vi "get filter mode.vi"(10 "filter rate":dbl, 11 "Numeric in":u32) -> (2 "filter mode":i32, 3 "no fit filter":bool)   [LabVIEW 2021]
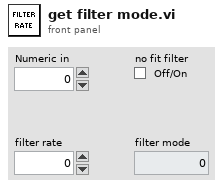
[diagram p1: front panel]
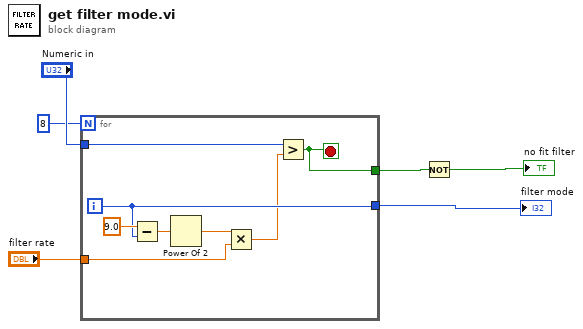
[diagram p0: block diagram]
diagram:
  n1 = for {
    N: 8 -> [_]
    tunnel: "Numeric in" -> [w14]
    tunnel: [w10] -> w4
    tunnel: [w13] -> w2
    tunnel: "filter rate" -> [w7]
    i -> [w10]
    stop <- w13 stop-if-true
    n2 = Subtract(x=9.0, y=w10) -> (x-y=w9:dbl)
    n3 = Power Of 2(x=w9) -> (2^x=w12:dbl)
    n4 = Multiply(x=w12, y=w7) -> (x*y=w8:dbl)
    n5 = Greater?(x=w14, y=w8) -> (0:w13:bool)
  }
  "filter mode" <- w4
  n6 = Not(x=w2) -> (.not. x?=→"no fit filter":bool)
